vi "Sound Sensor.vi"() -> ()   [LabVIEW 2017]
uses:
  <vilib>/DAQmx/read.llb/DAQmx Read (Analog 1D DBL 1Chan NSamp).vi
  <vilib>/DAQmx/miscellaneous.llb/DAQmx Fill In Error Info.vi
panel:
  out "Waveform Chart":dbl[](graph)
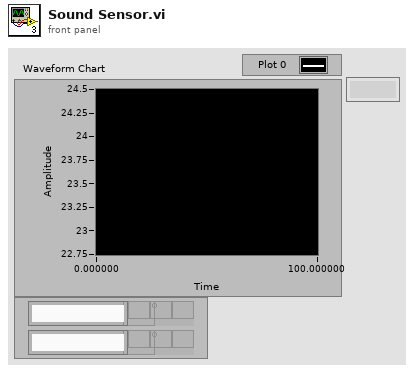
[diagram p1: front panel]
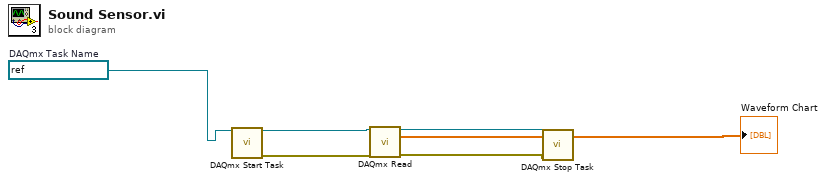
[diagram p0: block diagram]
diagram:
  w4 = refnum<k21> "Sound Sensor"  # DAQmx Task Name
  n1 = call <vilib>:"DAQmx Start Task.vi"("task/channels in"=w4) -> ("task out"=w3:refnum<k21>, "error out"=w6:errorcluster)  [unwired: 13 in]
  n2 = call-poly <vilib>:"DAQmx Read.vi"("task/channels in"=w3, "error in"=w6) -> ("task out"=w2:refnum<k21>, "data"=→"Waveform Chart":dbl[], "error out"=w5:errorcluster)  [unwired: 11 in]
  n3 = call <vilib>:"DAQmx Stop Task.vi"("task/channels in"=w2, "error in"=w5) -> ()  [unwired: 12 in, 2 out]
